vi "ReadTDMSTest.vi"() -> ()   [LabVIEW 2020]
panel:
  out "Waveform Graph 3":dbl[](graph)
  out "Waveform Graph 2":dbl[](graph)
  out "Waveform Graph":dbl[](graph)
  out "channel name(s) out":string[](array[string])
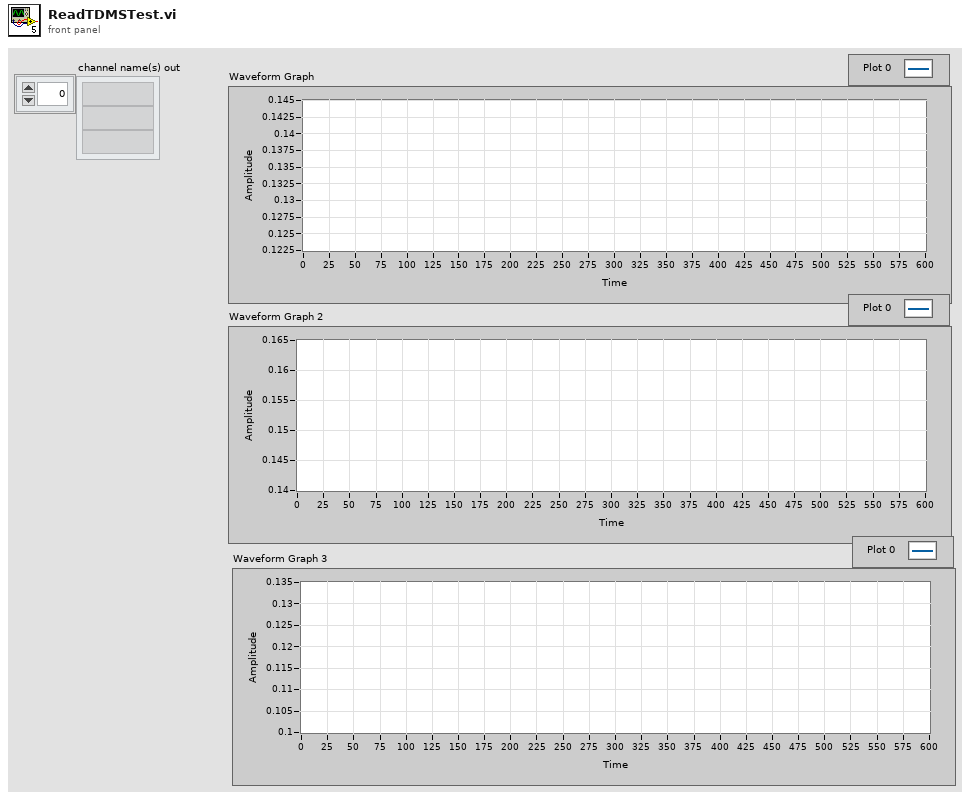
[diagram p1: front panel]
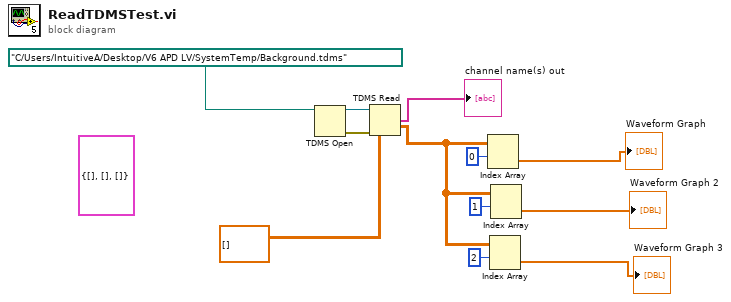
[diagram p0: block diagram]
diagram:
  (unwired) cluster{dbl[], dbl[], dbl[]} {[], [], []}
  n1 = TDMS Open(11:path "C:/Users/IntuitiveA/Desktop/V6 APD LV/SystemTemp/Background.tdms") -> (0:w11:errorcluster, 3:w12:refnum<k34>)  [unwired: 6 in]
  n2 = TDMS Read(0:w12, 11:w11, 12:dbl[][] []) -> (8:→"channel name(s) out":string[], 10:w5:dbl[][])  [unwired: 5 in, 4 out]
  n3 = Index Array(array=w5, index (row)=0) -> (element=→"Waveform Graph":dbl[])  [unwired: 1 in]
  n4 = Index Array(array=w5, index (row)=2) -> (element=→"Waveform Graph 3":dbl[])  [unwired: 1 in]
  n5 = Index Array(array=w5, index (row)=1) -> (element=→"Waveform Graph 2":dbl[])  [unwired: 1 in]
